vi "Construct Command.vi"(10 "Channel":u16, 11 "HH802U in":refnum<class "HH802U.lvclass">) -> (2 "CMD":string, 3 "HH802U out":refnum<class "HH802U.lvclass">)   [LabVIEW 2015, in "HH802U.lvclass"]
uses:
  HH802U.lvclass
  HH802U.lvclass/HH802U.ctl
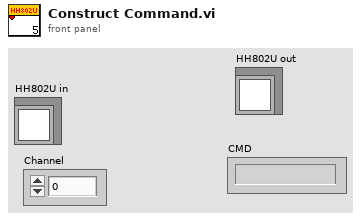
[diagram p1: front panel]
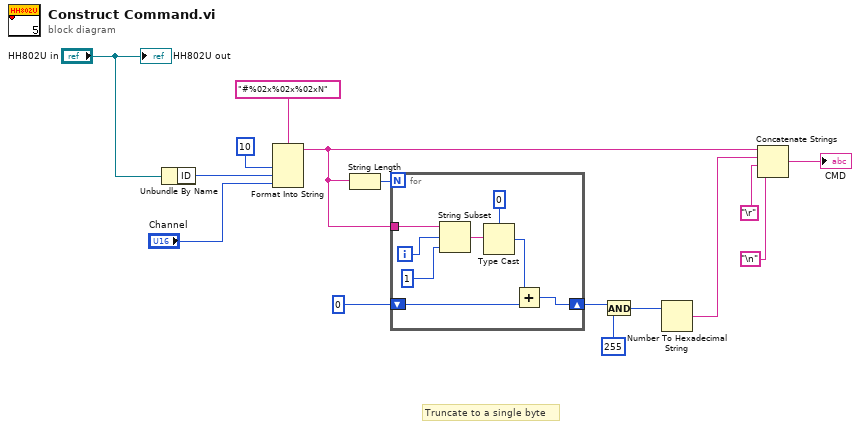
[diagram p0: block diagram]
diagram:
  # "Truncate to a single byte"
  n1 = Unbundle By Name("HH802U in") -> ("ID"=w3:u16)
  n2 = Format Into String(format string="#%02x%02x%02xN", 10 ("Command Length"), w3, "Channel") -> (resulting string=w2:string)  [unwired: 2 in, 1 out]
  n3 = String Length(string=w2) -> (length=w7:i32)
  n4 = for {
    N: w7 -> [_]
    tunnel: w2 -> [w23]
    shift-right: [w18] -> w9
    shift-left: u16 0 ("width (-)") -> [w19]
    i -> [w22]
    n5 = String Subset(string=w23, offset (0)=w22, length (rest)=1 ("length (rest)")) -> (substring=w20:string)
    n6 = Type Cast(type=u8 0 ("output 2"), x=w20) -> (*(type *) &x=w17:u8)
    n7 = Add(x=w17, y=w19) -> (x+y=w18:u16)
  }
  n8 = And(x=w9, y=u16 255) -> (x .and. y?=w11:u16)
  n9 = Number To Hexadecimal String(2:w11) -> (0:w12:string)  [unwired: 1 in]
  n10 = Concatenate Strings(w2, w12, "\r", "\n") -> (→"CMD":string)
  "HH802U out" <- "HH802U in"
